vi "SWLDA.vi"(5 "premove":dbl=0.5, 7 "penter":dbl=0.4, 8 "Maximum_Iteration":dbl=88.0, 10 "ERP_Nontarget":dbl[][](array[numeric]) format="%0.3f", 11 "ERP_Target":dbl[][](array[numeric]) format="%0.3f") -> (2 "WEIGHT":dbl[](array[numeric]), 3 "LDA_matrix":T1)   [LabVIEW 2014]
uses:
  <vilib>/Analysis/Matrix/Datatypes/RealMatrix.ctl
  <vilib>/Analysis/baseanly.llb/Vector x A.vi
  <vilib>/Analysis/Matrix/Numeric/Conversions/Array To Matrix - RA.vi
  <vilib>/Analysis/Matrix/Numeric/Conversions/Array To Matrix - RA2.vi
  <vilib>/Analysis/NI_AALBase.lvlib
  <vilib>/Analysis/Matrix/NI_Matrix.lvlib
panel:
  out "biase":dbl[](array[numeric])
  out "Nontarget_mean":dbl[](array[numeric])
  out "Target_mean":dbl[](array[numeric])
  out "Label":dbl[](array[numeric])
  out "in":dbl[](array[numeric])
  out "Weight":dbl[](array[numeric])
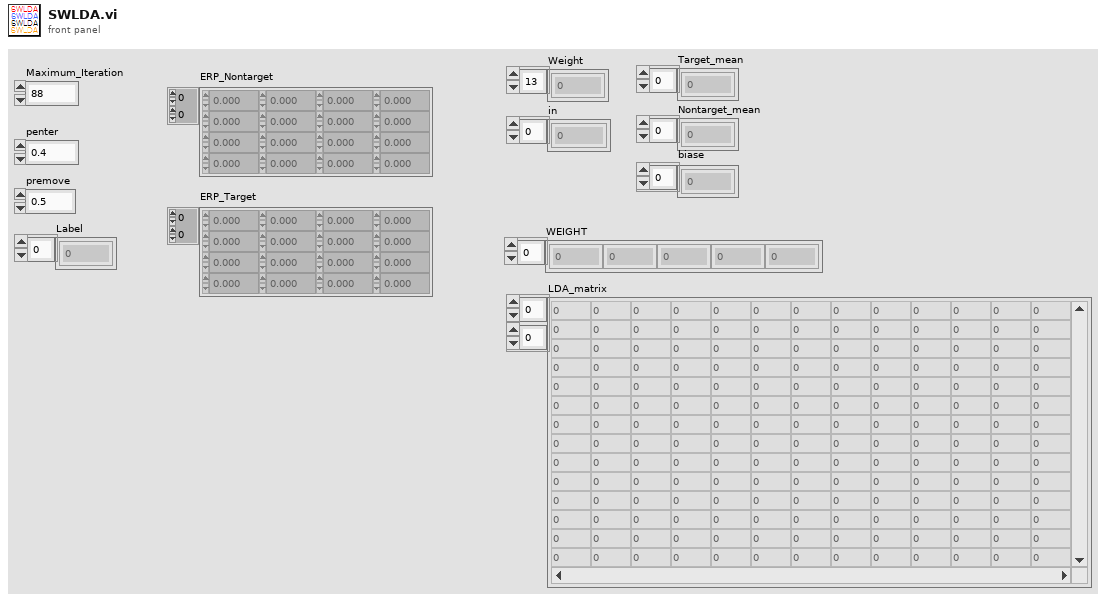
[diagram p1: front panel]
types:
  T1 = typedef "NI_Matrix.lvlib/RealMatrix.ctl" = dbl[][]
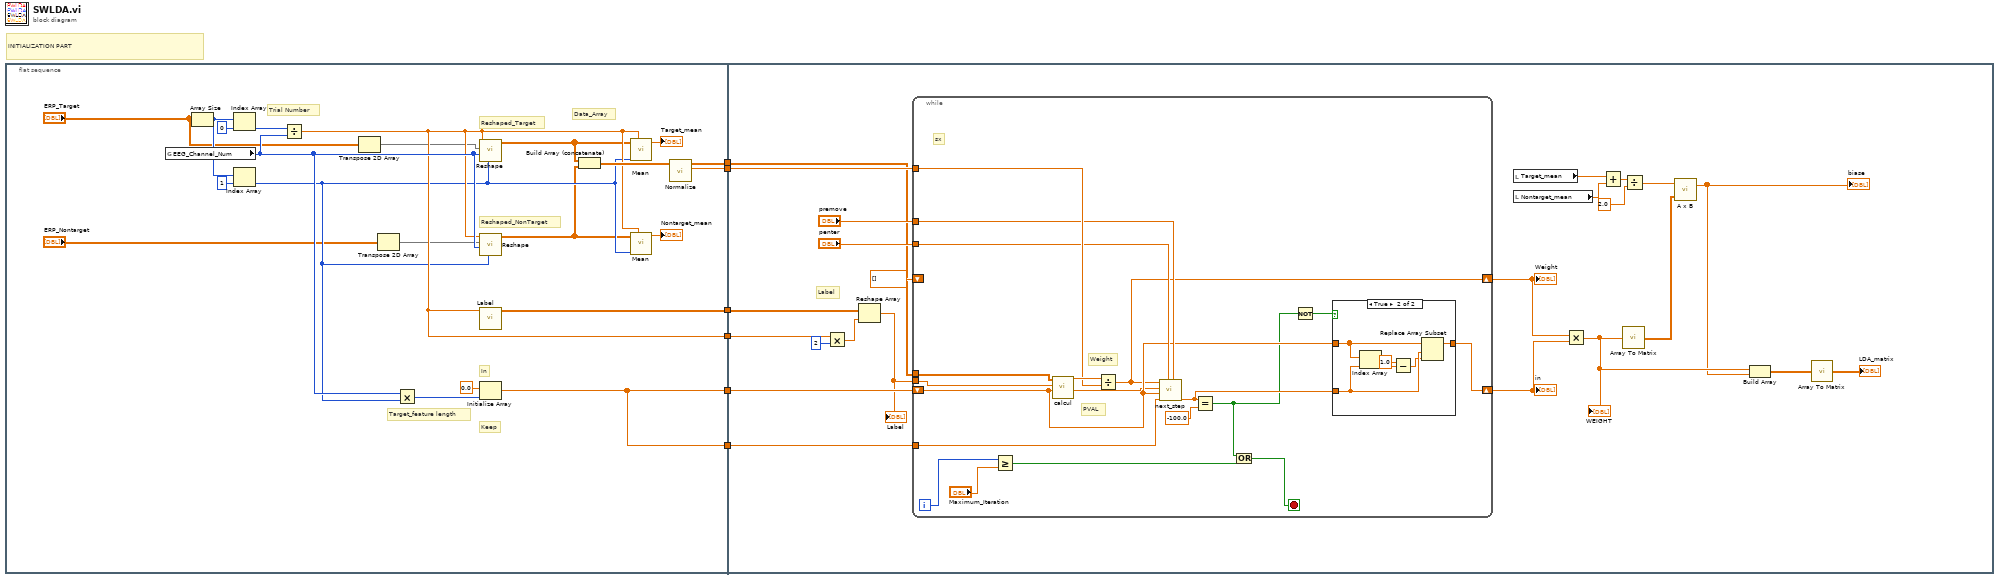
[diagram p0: block diagram]
diagram:
  # "INITIALIZATION PART"
  n1 = flat-sequence {
    tunnel: [w17] -> w6
    tunnel: [w17] -> w5
    tunnel: [w21] -> w4
    tunnel: [w20] -> w3
    tunnel: [w19] -> w2
    tunnel: [w15] -> w1
    tunnel: w6 -> [w51]
    tunnel: w5 -> [w46]
    tunnel: w4 -> [w52]
    tunnel: w3 -> [w42]
    tunnel: w2 -> [w49]
    tunnel: w1 -> [w41]
    frame #0 {
      # "Keep"
      # "In"
      # "Target_feature length"
      # "Data_Array"
      # "Reshaped_NonTarget"
      # "Reshaped_Target"
      # "Trial Number"
      n2 = global read "Control_Panel.vi" "EEG_Channel_Num"() -> (w24:i32)
      n3 = Array Size(array="ERP_Target") -> (size(s)=w26:i32[])
      n4 = Index Array(array=w26, index=0) -> (element=w25:i32)
      n5 = Index Array(array=w26, index=1) -> (element=w14:i32)
      n6 = Divide(x=w25, y=w24) -> (x/y=w15:dbl)
      n7 = Transpose 2D Array(2D array="ERP_Target") -> (transposed array=w12:dbl[][])
      n8 = Transpose 2D Array(2D array="ERP_Nontarget") -> (transposed array=w11:dbl[][])
      n9 = Multiply(x=w24, y=w14) -> (x*y=w23:i32)
      n10 = call "Reshape.vi"("Numeric"=w14, "EEG_Channel_Num"=w24, "all rows"=w12, "Numeric 2"=w15) -> ("Array"=w9:dbl[][])  [unwired: 7 in]
      n11 = call "Reshape.vi"("Numeric"=w14, "EEG_Channel_Num"=w24, "all rows"=w11, "Numeric 2"=w15) -> ("Array"=w10:dbl[][])  [unwired: 7 in]
      n12 = call "Label.vi"("Numeric"=w15) -> ("Array"=w21:dbl[][])  [unwired: 10 in]
      n13 = Initialize Array(0.0 ("element"), w23) -> (w17:dbl[])
      n14 = Build Array (concatenate)(w9, w10) -> (w18:dbl[][])
      n15 = call "Mean.vi"("trial_number"=w15, "feature_number"=w14, "Target/NonTarget"=w9) -> ("mean"=→"Target_mean":dbl[])  [unwired: 8 in]
      n16 = call "Mean.vi"("trial_number"=w15, "feature_number"=w14, "Target/NonTarget"=w10) -> ("mean"=→"Nontarget_mean":dbl[])  [unwired: 8 in]
      n17 = call "Normalize.vi"("Data"=w18) -> ("sx"=w19:dbl[], "Data_out"=w20:dbl[][])  [unwired: 8 in, 1 out]
    }
    frame #1 {
      # "Label"
      n18 = Multiply(x=w41, y=2) -> (x*y=w44:dbl)
      n19 = Reshape Array(w52, w44) -> (w50:dbl[])
      "Label" <- w50
      n20 = while {
        shift-right: [w58] -> w35
        shift-left: w51 -> [w59]
        tunnel: w50 -> [w67]
        tunnel: w42 -> [w66]
        tunnel: w49 -> [w64]
        tunnel: "penter" -> [w63]
        tunnel: "premove" -> [w62]
        tunnel: w46 -> [w61]
        shift-right: [w57] -> w36
        shift-left: dbl[] [] -> [_]
        i -> [w71]
        stop <- w68 stop-if-true
        # "sx"
        # "PVAL"
        # "Weight"
        n21 = Greater Or Equal?(x=w71, y="Maximum_Iteration") -> (x >= y?=w69:bool)
        n22 = call "calcul.vi"("In"=w59, "Label (y)"=w67, "Data (allx)"=w66) -> ("PVAL"=w53:dbl[], "B"=w65:dbl[])  [unwired: 7 in]
        n23 = Divide(x=w65, y=w64) -> (x/y=w57:dbl[])
        n24 = call "next_step.vi"("premove"=w62, "penter"=w63, "keep"=w61, "in"=w59, "PVal"=w53, "B"=w57) -> ("swap"=w56:dbl)  [unwired: 4 in, 1 out]
        n25 = Equal?(x=w56, y=-100.0) -> (x = y?=w54:bool)
        n26 = Or(x=w54, y=w69) -> (x .or. y?=w68:bool)
        n27 = Not(x=w54) -> (.not. x?=w55:bool)
        n28 = case shown="True" w55 {
          tunnel: w59 -> [w72 w77]
          tunnel: w56 -> [_ w76]
          tunnel: [w72 w78] -> w58
          frame False {
          }
          frame True {
            n29 = Index Array(array=w77, index=w76) -> (element=w75:dbl)
            n30 = Subtract(x=1.0, y=w75) -> (x-y=w73:dbl)
            n31 = Replace Array Subset(array=w77, new element=w73, index=w76) -> (w78:dbl[])
          }
        }
      }
      "Weight" <- w36
      "in" <- w35
      n32 = local read "Target_mean"() -> (w40:dbl[])
      n33 = local read "Nontarget_mean"() -> (w39:dbl[])
      n34 = Multiply(x=w36, y=w35) -> (x*y=w30:dbl[])
      "WEIGHT" <- w30
      n35 = Add(x=w40, y=w39) -> (x+y=w38:dbl[])
      n36 = call-poly <vilib>:"Array To Matrix.vi"("Real 1D Array"=w30) -> ("Real Matrix (Column Vector)"=w33:T1)
      n37 = Divide(x=w38, y=2.0) -> (x/y=w34:dbl[])
      n38 = call-poly <vilib>:"A x B.vi"("Matrix A"=w33, "Vector V'"=w34) -> ("V' x A"=w29:dbl[])  [unwired: 1 out]
      "biase" <- w29
      n39 = Build Array(w30, w29) -> (w31:dbl[][])
      n40 = call-poly <vilib>:"Array To Matrix.vi"("Real 2D Array"=w31) -> ("Real Matrix"=→"LDA_matrix":T1)
    }
  }
